vi "pwm period set.vi"(10 "PWM frequence":dbl) -> (0 "pwm cnfg":T1)   [LabVIEW 2019, in "my FPGA lib.lvlib" / "motor.lvlib"]
uses:
  motor.lvlib
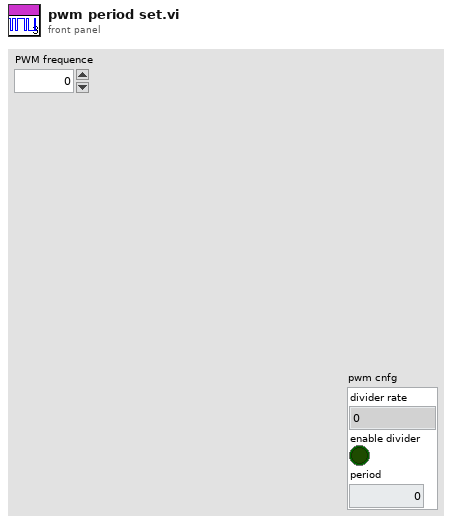
[diagram p1: front panel]
types:
  T1 = cluster{"divider rate":i32, "enable divider":bool, "period":i32}
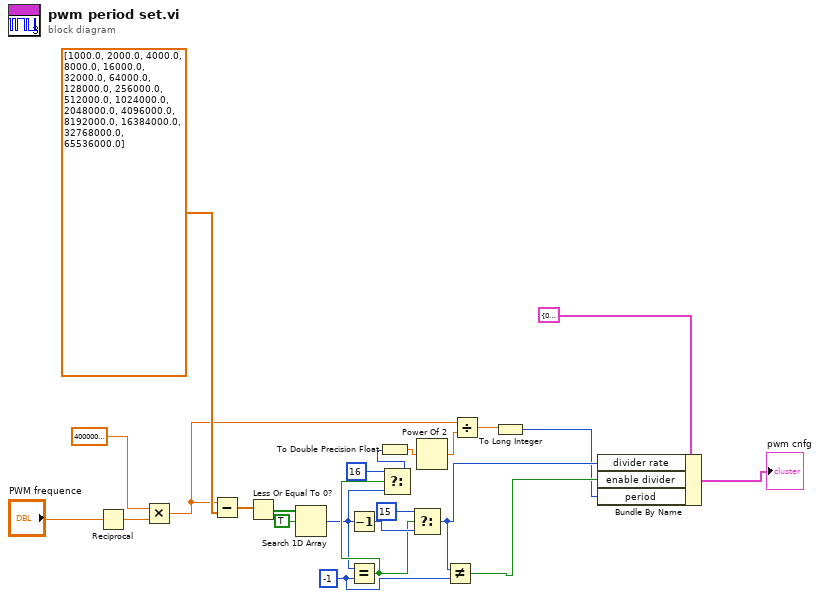
[diagram p0: block diagram]
diagram:
  w15 = -1 ("y")
  n1 = Reciprocal(x="PWM frequence") -> (1/x=w22:dbl)
  n2 = Multiply(x=40000000.0, y=w22) -> (x*y=w14:dbl)
  n3 = Subtract(x=w14, y=dbl[] [1000.0, 2000.0, 4000.0, 8000.0, 16000.0, 32000.0, 64000.0, 128000.0, 256000.0, 512000.0, 1024000.0, 2048000.0, 4096000.0, 8192000.0, 16384000.0, 32768000.0, 65536000.0]) -> (x-y=w19:dbl[])
  n4 = Less Or Equal To 0?(x=w19) -> (x <= 0?=w18:bool[])
  n5 = Search 1D Array(1D array=w18, element=TRUE) -> (index of element=w11:i32)  [unwired: 1 in]
  n6 = Decrement(x=w11) -> (x-1=w16:i32)
  n7 = Equal?(x=w11, y=w15) -> (x = y?=w13:bool)
  n8 = Select(t=16, s=w13, f=w11) -> (s? t:f=w9:i32)
  n9 = To Double Precision Float(number=w9) -> (double precision float=w8:dbl)
  n10 = Select(t=15, s=w13, f=w16) -> (s? t:f=w3:i32)
  n11 = Power Of 2(x=w8) -> (2^x=w7:dbl)
  n12 = Not Equal?(x=w3, y=w15) -> (x != y?=w4:bool)
  n13 = Divide(x=w14, y=w7) -> (x/y=w6:dbl)
  n14 = To Long Integer(number=w6) -> (32bit integer=w2:i32)
  n15 = Bundle By Name(cluster=T1 {"divider rate"=0, "enable divider"=FALSE, "period"=0} ("pwm cnfg"), "divider rate"=w3, "enable divider"=w4, "period"=w2) -> (→"pwm cnfg":T1)
